vi "VI Under Test.vi"() -> ()   [LabVIEW 2020, in "Template Test Vector.lvclass"]
uses:
  Template Test Vector.lvclass
panel:
  out "Indicator name":string
  in  "Control name":string
  # "This is a dummy VI for demonstration purpose."
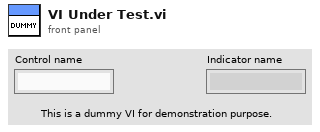
[diagram p1: front panel]
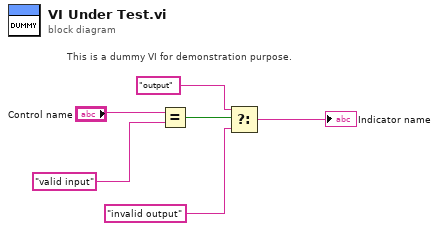
[diagram p0: block diagram]
diagram:
  # "This is a dummy VI for demonstration purpose."
  n1 = Equal?(x="Control name", y="valid input" ("Control Name")) -> (x = y?=w3:bool)
  n2 = Select(t="output" ("Control Name"), s=w3, f="invalid output" ("Control Name")) -> (s? t:f=→"Indicator name":string)
